vi "Get Packet Type (TCP Packet).vi"(8 "Error In":errorcluster, 9 "Ctl index":u8, 10 "TCP/IP Data in":u8[](array[numeric])) -> (0 "Error Out":errorcluster, 2 "TCP/IP Data out":u8[](array[numeric]), 3 "Return Packet Type":T1)   [LabVIEW 2014, in "hse-db.lvlib" / "MySQL (TCP).lvlib"]
uses:
  MySQL (TCP).lvlib
  Controls/Return Packet Types.ctl
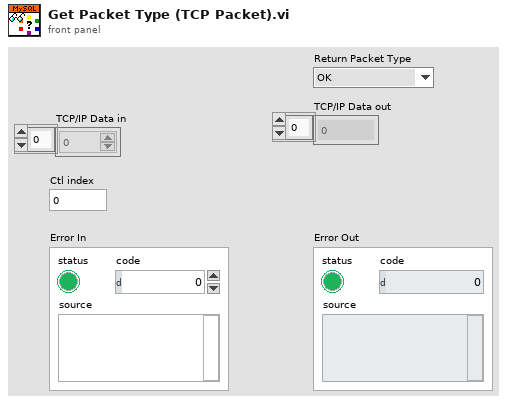
[diagram p1: front panel]
types:
  T1 = typedef "hse-db.lvlib/MySQL (TCP).lvlib/Return Packet Types.ctl" = enum16{"OK", "Result Set Header", "Error", "Field", "Row", "EOF"}
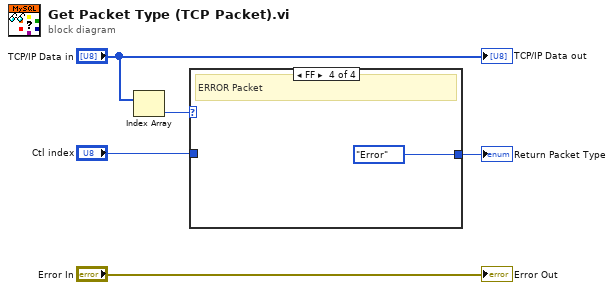
[diagram p0: block diagram]
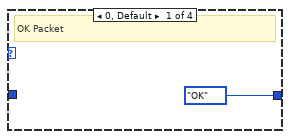
[diagram p2: hidden frame]
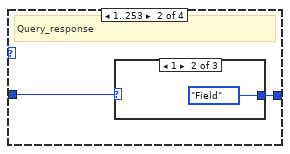
[diagram p3: hidden frame]
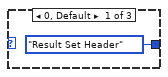
[diagram p4: hidden frame]
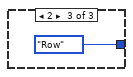
[diagram p5: hidden frame]
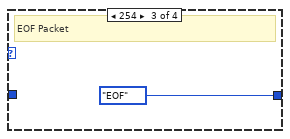
[diagram p6: hidden frame]
diagram:
  n1 = Index Array(array="TCP/IP Data in") -> (element=w4:u8)  [unwired: 1 in]
  n2 = case shown="FF" w4 {
    tunnel: [Return_Packet_Types."OK" ("Previous Packet Type 2") w8 Return_Packet_Types."EOF" ("Previous Packet Type 2") Return_Packet_Types."Error" ("Previous Packet Type 2")] -> w3
    tunnel: "Ctl index" -> [_ w7 _ _]
    frame 0, Default {
      # "OK Packet"
    }
    frame 1..253 {
      # "Query_response"
      n3 = case shown="1" w7 {
        tunnel: [Return_Packet_Types."Result Set Header" ("Previous Packet Type 2") Return_Packet_Types."Field" ("Previous Packet Type 2") Return_Packet_Types."Row" ("Previous Packet Type 2")] -> w8
        frame 0, Default {
        }
        frame 1 {
        }
        frame 2 {
        }
      }
    }
    frame 254 {
      # "EOF Packet"
    }
    frame 255 {
      # "ERROR Packet"
    }
  }
  "Return Packet Type" <- w3
  "TCP/IP Data out" <- "TCP/IP Data in"
  "Error Out" <- "Error In"
